vi "Get Enable Rmb User.vi"(5 "[Data] Recent User in":refnum<class "[Data] Recent User.lvclass">) -> (2 "enable rmb user":bool)   [LabVIEW 2020, in "[Data] Recent User.lvclass"]
uses:
  [Data] Recent User.lvclass
  [Data] Recent User.lvclass/[Data] Recent User.ctl
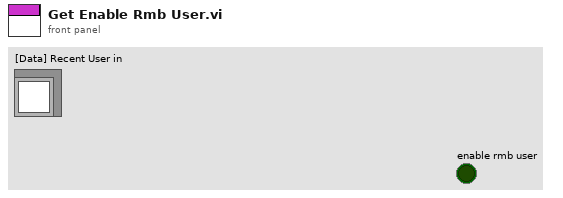
[diagram p1: front panel]
types:
  T1 = cluster{"enable rmb user":bool, "recent user list":string[]}
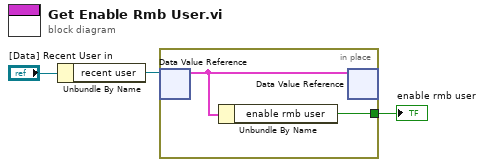
[diagram p0: block diagram]
diagram:
  n1 = Unbundle By Name("[Data] Recent User in") -> ("recent user"=w1:refnum<data-value>)
  n2 = in-place {
    in-place-border: [w4] -> w2
    n3 = in-place-dvr #1(w1) -> (w5:T1)  [unwired: 1 out]
    n4 = Unbundle By Name(w5) -> ("enable rmb user"=w4:bool)
    n5 = in-place-dvr #1(w5) -> ()  [unwired: 2 out]
  }
  "enable rmb user" <- w2
